vi "VisionPositionControlAngleToSpeaker.vi"(11 "TargetAngle":dbl) -> (2 "OnTargetSpeaker":bool, 3 "DesiredAngularSpeed (degree/s)":dbl)   [LabVIEW 2023]
doc: "Position control for angle to speaker\ninputs:\n--TargetPosition--degrees--Numeric--(probably use VisionGetDistanceAndAngleToSpeaker)\noutputs:\n--DesiredSpeed--degrees/s--Numeric\n--OnTarget--boolean"
uses:
  <vilib>/Rock Robotics/WPI/ThirdParty/JAS_Junk/TrajLib/MathUtil_Clamp.vi
  <vilib>/Rock Robotics/WPI/ThirdParty/JAS_Junk/TrajLib/Rotation2d_GetRadians.vi
  <vilib>/Rock Robotics/WPI/ThirdParty/JAS_Junk/TrajLib/Conv_Radians_Deg.vi
  VisionGlobal.vi
  <vilib>/Rock Robotics/WPI/ThirdParty/JAS_Junk/TrajLib/Trajectory_Library.lvlib
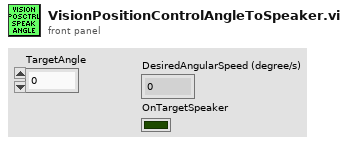
[diagram p1: front panel]
types:
  T1 = typedef "Trajectory_Library.lvlib/POSE2D.ctl" = cluster{"TRANSLATION":T2, "ROTATION":T3}
  T2 = typedef "Trajectory_Library.lvlib/TRANSLATION2D.ctl" = cluster{"X":dbl, "Y":dbl}
  T3 = typedef "Trajectory_Library.lvlib/ROTATION2D.ctl" = cluster{"VALUE":dbl, "COS":dbl, "SIN":dbl}
  T4 = typedef "Trajectory_Library.lvlib/PosCtrl_Tuning_Type.ctl" = cluster{"Slope":dbl, "Offset":dbl, "Error Deadband":dbl, "At Reference Count":i32, "Negate Output":bool, "Max Allowd Position":dbl, "Min Allowd Position":dbl}
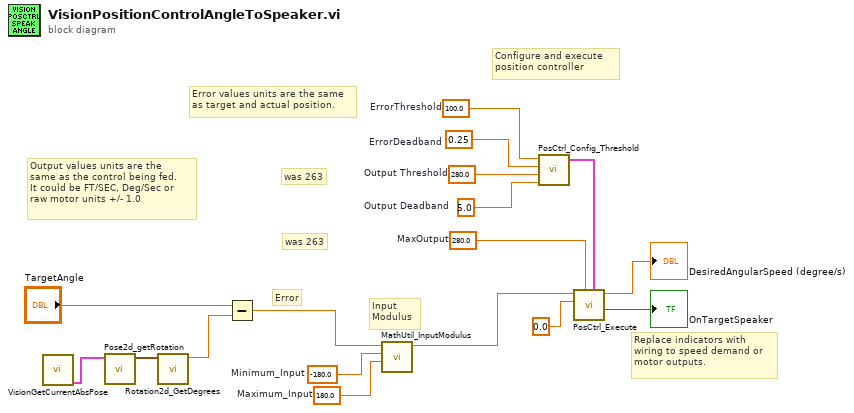
[diagram p0: block diagram]
diagram:
  w4 = -180.0  # Minimum_Input
  w3 = 180.0  # Maximum_Input
  w17 = 280.0  # MaxOutput
  w13 = 100.0  # ErrorThreshold
  w12 = 0.25  # ErrorDeadband
  w11 = 280.0  # Output Threshold
  w10 = 5.0  # Output Deadband
  # "was 263"
  # "was 263"
  # "Error"
  # "Input\nModulus"
  # "Replace indicators with\nwiring to speed demand or\nmotor outputs."
  # "Output values units are the\nsame as the control being fed.  \nIt could be FT/SEC, Deg/Sec or\nraw motor units +/- 1.0"
  # "Error values units are the same \nas target and actual position."
  # "Configure and execute \nposition controller"
  n1 = call "VisionGetCurrentAbsPose.vi"() -> ("Current ABS Pose"=w8:T1)  [unwired: 9 in]
  n2 = call <vilib>:"Pose2d_getRotation.vi"("in POSE"=w8) -> ("out ROTATION"=w9:T3)  [unwired: 10 in]
  n3 = call <vilib>:"Rotation2d_GetDegrees.vi"("in ROTATION"=w9) -> ("AngleDegrees"=w5:dbl)  [unwired: 10 in]
  n4 = Subtract(x="TargetAngle", y=w5) -> (x-y=w2:dbl)
  n5 = call <vilib>:"MathUtil_InputModulus.vi"("Maximum_Input"=w3, "Minimum_Input"=w4, "Input"=w2) -> ("modulus"=w1:dbl)  [unwired: 8 in]
  n6 = call <vilib>:"PosCtrl_Config_Threshold.vi"("Output Deadband"=w10, "Output Threshold"=w11, "ErrorDeadband"=w12, "ErrorThreshold"=w13) -> ("PosCtrl_Config_Params"=w14:T4)  [unwired: 7 in]
  n7 = call <vilib>:"PosCtrl_Execute.vi"("PosCtrl_Config_Params"=w14, "MaxOutput"=w17, "CurrentPosition"=0.0, "TargetPosition"=w1) -> ("OnTarget"=→"OnTargetSpeaker":bool, "Output"=→"DesiredAngularSpeed (degree/s)":dbl)  [unwired: 5 in, 1 out]
